vi "Lockin.vi"(10 "Config":T1={"Ref channel index"=1, "Active channel index"=2}, 11 "array":waveform(dbl)[](array[waveform])) -> (2 "Output waveform":waveform(dbl)[](array[waveform]), 3 "Lockin output":T2 {"X" format="%#_3g"; "Y" format="%#_3g"; "R" format="%#_3g"})   [LabVIEW 2019]
doc: "This example demonstrates how to acquire a continuous amount of data (Waveform) using the DAQ device's internal clock. It also shows how to synchronize two devices for different device families (E Series, S Series, M Series, X Series, DSA, and SC Express), to simultaneously acquire the data.\n\nFor instructions on how to connect your signals to the DAQ device, refer to your device documentation."
uses:
  <vilib>/Waveform/WDTOps.llb/WDT Get Final Time Value DBL.vi
  <vilib>/Analysis/NI_AALPro.lvlib
panel:
  out "Ref waveform":waveform(dbl)[](array[waveform])
  # "Lockin"
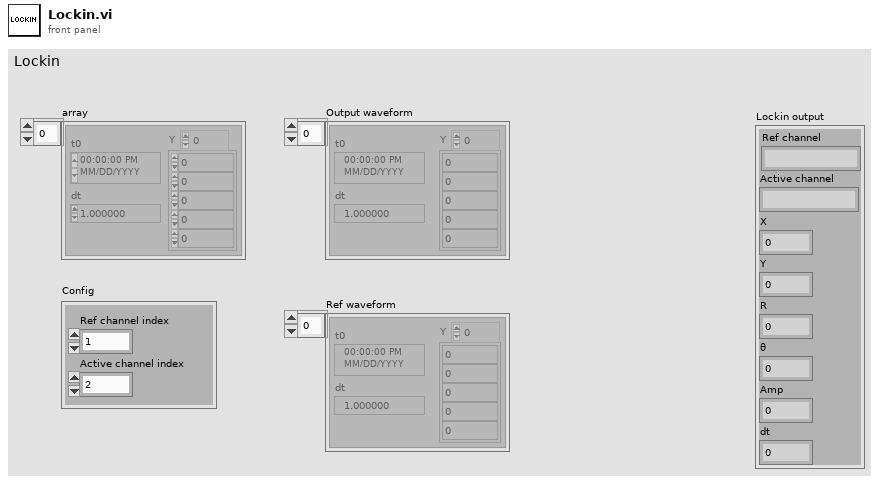
[diagram p1: front panel]
types:
  T1 = cluster{"Ref channel index":i32, "Active channel index":i32}
  T2 = cluster{"X":dbl, "Y":dbl, "R":dbl, "θ":dbl, "Amp":dbl, "dt":dbl, "Active channel":string, "Ref channel":string}
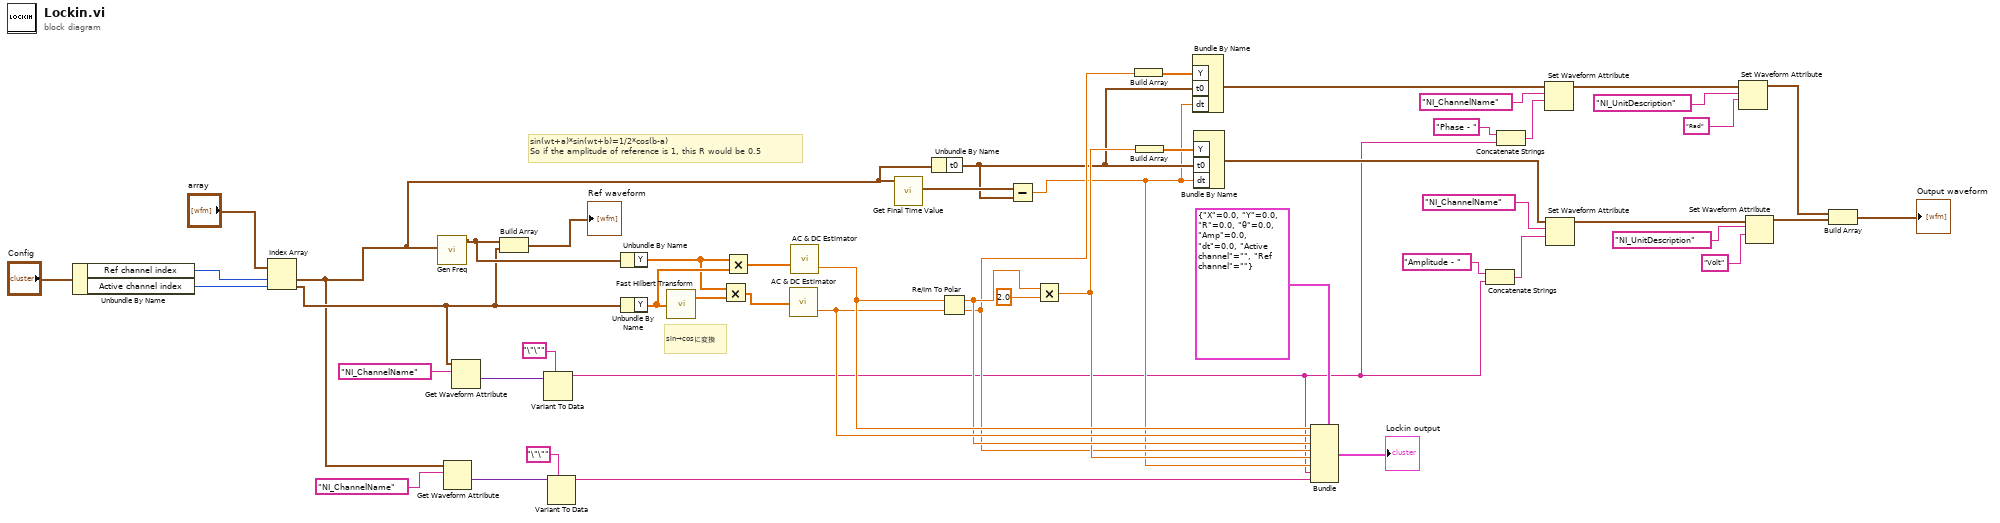
[diagram p0: block diagram]
diagram:
  # "sin(wt+a)*sin(wt+b)=1/2*cos(b-a)\nSo if the amplitude of reference is 1, this R would be 0.5"
  # "sin→cosに変換"
  n1 = Unbundle By Name("Config") -> ("Ref channel index"=w5:i32, "Active channel index"=w4:i32)
  n2 = Index Array(array="array", index #1=w5, index #2=w4) -> (element #1=w9:waveform(dbl), element #2=w15:waveform(dbl))
  n3 = call "Gen Freq.vi"("Ref"=w9) -> ("Ref_PLL_Out"=w45:waveform(dbl))  [unwired: 10 in]
  n4 = Get Waveform Attribute(6:"NI_ChannelName" ("name"), 7:w9) -> (1:w7:variant)  [unwired: 2 in, 3 out]
  n5 = Get Waveform Attribute(6:"NI_ChannelName" ("name"), 7:w15) -> (1:w13:variant)  [unwired: 2 in, 3 out]
  n6 = Build Array(w45, w15) -> (→"Ref waveform":waveform(dbl)[])
  n7 = Variant To Data(type="\"\"" ("name"), Variant=w13) -> (data=w2:string)  [unwired: 1 in, 1 out]
  n8 = Variant To Data(type="\"\"" ("name"), Variant=w7) -> (data=w1:string)  [unwired: 1 in, 1 out]
  n9 = Unbundle By Name(w45) -> ("Y"=w49:dbl[])
  n10 = Unbundle By Name(w15) -> ("Y"=w50:dbl[])
  n11 = call <vilib>:"Fast Hilbert Transform.vi"("X"=w50) -> ("Hilbert{X}"=w51:dbl[])  [unwired: 1 out]
  n12 = Multiply(x=w49, y=w51) -> (x*y=w47:dbl[])
  n13 = Multiply(x=w49, y=w50) -> (x*y=w48:dbl[])
  n14 = call <vilib>:"AC & DC Estimator.vi"("Signal (V)"=w47) -> ("DC estimate (V)"=w43:dbl)  [unwired: 1 out]
  n15 = call <vilib>:"AC & DC Estimator.vi"("Signal (V)"=w48) -> ("DC estimate (V)"=w44:dbl)  [unwired: 1 out]
  n16 = call-poly <vilib>:"Get Final Time Value.vi"("waveform in"=w9) -> ("tf"=w38:timestamp)  [unwired: 8 in, 2 out]
  n17 = Unbundle By Name(w9) -> ("t0"=w34:timestamp)
  n18 = Re/Im To Polar(2:w43, 3:w44) -> (0:w35:dbl, 1:w42:dbl)
  n19 = Subtract(x=w38, y=w34) -> (x-y=w11:dbl)
  n20 = Multiply(x=w42, y=2.0) -> (x*y=w40:dbl)
  n21 = Build Array(w35) -> (w36:dbl[])
  n22 = Build Array(w40) -> (w41:dbl[])
  n23 = Bundle By Name("Y"=w36, "t0"=w34, "dt"=w11) -> (w31:waveform(dbl))  [unwired: 1 in]
  n24 = Bundle By Name("Y"=w41, "t0"=w34, "dt"=w11) -> (w30:waveform(dbl))  [unwired: 1 in]
  n25 = Bundle(cluster=T2 {"X"=0.0, "Y"=0.0, "R"=0.0, "θ"=0.0, "Amp"=0.0, "dt"=0.0, "Active channel"="", "Ref channel"=""} ("Lock-in output"), "X"=w44, "Y"=w43, "R"=w42, "θ"=w35, "Amp"=w40, "dt"=w11, "Active channel"=w2, "Ref channel"=w1) -> (→"Lockin output":T2)
  n26 = Concatenate Strings("Amplitude - " ("name"), w2) -> (w25:string)
  n27 = Concatenate Strings("Phase - " ("name"), w2) -> (w26:string)
  n28 = Set Waveform Attribute(5:w26, 6:"NI_ChannelName" ("name"), 7:w31) -> (3:w21:waveform(dbl))  [unwired: 1 in, 2 out]
  n29 = Set Waveform Attribute(5:w25, 6:"NI_ChannelName" ("name"), 7:w30) -> (3:w19:waveform(dbl))  [unwired: 1 in, 2 out]
  n30 = Set Waveform Attribute(5:"Rad" ("name"), 6:"NI_UnitDescription" ("name"), 7:w21) -> (3:w20:waveform(dbl))  [unwired: 1 in, 2 out]
  n31 = Set Waveform Attribute(5:"Volt" ("name"), 6:"NI_UnitDescription" ("name"), 7:w19) -> (3:w18:waveform(dbl))  [unwired: 1 in, 2 out]
  n32 = Build Array(w20, w18) -> (→"Output waveform":waveform(dbl)[])
